vi "InitDMs_DUAL.vi"(11 "BM Flats":bool) -> (2 "IDs":i32[](array[numeric]), 3 "reference out":refnum<k7>)   [LabVIEW 2014]
uses:
  <vilib>/Utility/file.llb/Read From Spreadsheet File (DBL).vi
  <vilib>/Utility/file.llb/Read From Spreadsheet File (string).vi
  <vilib>/Analysis/Matrix/Numeric/Conversions/Array To Matrix - RA2.vi
  <vilib>/Analysis/Matrix/NI_Matrix.lvlib
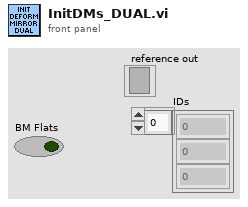
[diagram p1: front panel]
types:
  T1 = typedef "NI_Matrix.lvlib/RealMatrix.ctl" = dbl[][]
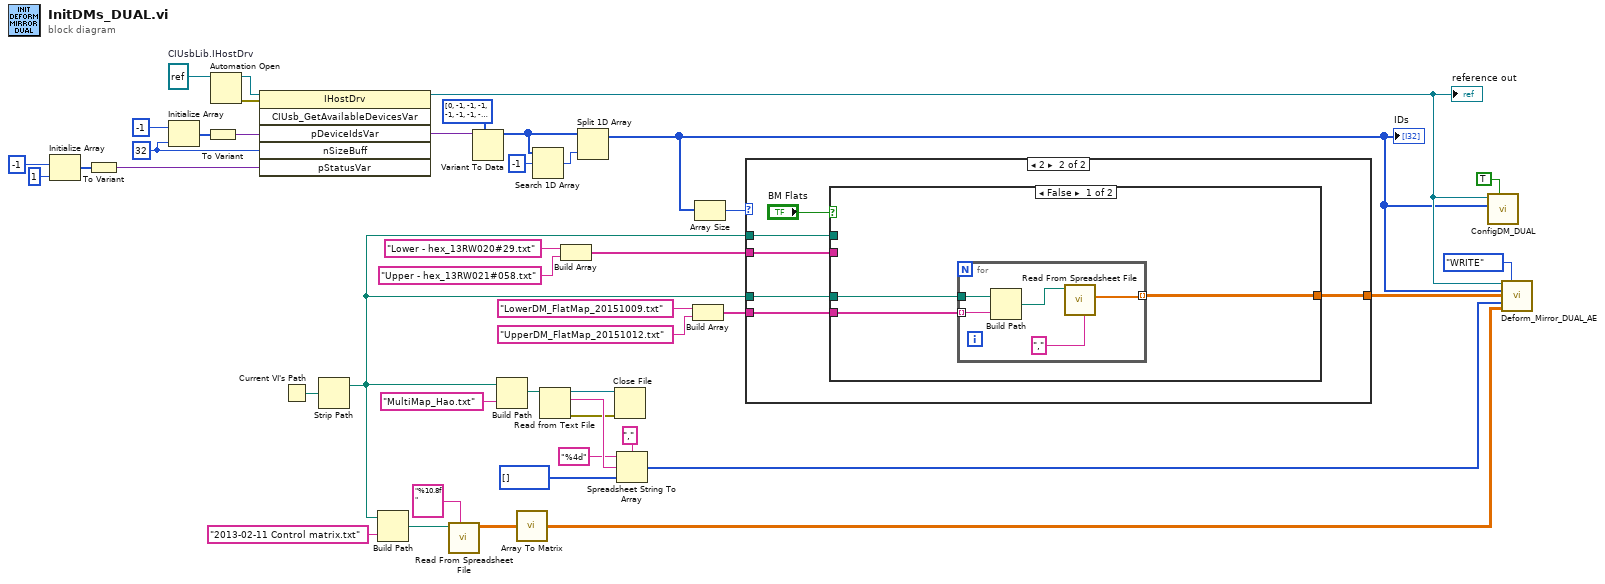
[diagram p0: block diagram]
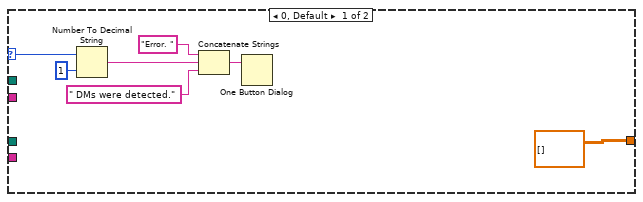
[diagram p2: hidden frame]
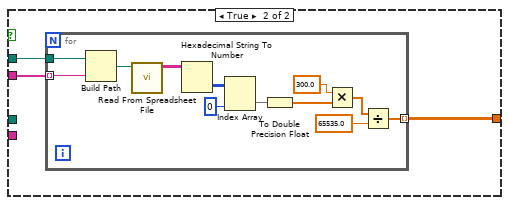
[diagram p3: hidden frame]
diagram:
  w39 = 32 ("dimension size")
  w31 = refnum<k7> refnum  # CIUsbLib.IHostDrv
  n1 = Initialize Array(-1 ("element"), 1 ("dimension size")) -> (w32:i32[])
  n2 = To Variant(anything=w32) -> (Variant=w38:variant)
  n3 = Initialize Array(-1 ("element"), w39) -> (w33:i32[])
  n4 = To Variant(anything=w33) -> (Variant=w34:variant)
  n5 = Automation Open(Automation Refnum=w31) -> (Automation Refnum=w7:refnum<k7>, error out=w36:errorcluster)  [unwired: 1 in, 2 out]
  n6 = invoke class="IHostDrv" method="CIUsb_GetAvailableDevicesVar"(reference=w7, error in=w36, "pDeviceIdsVar"=w34, "nSizeBuff"=w39, "pStatusVar"=w38) -> (reference out=w10:refnum<k7>, "pDeviceIdsVar"=w44:variant)  [unwired: 1 in, 4 out]
  "reference out" <- w10
  n7 = Current VI's Path() -> (path=w26:path)
  n8 = Strip Path(path=w26) -> (stripped path=w6:path)  [unwired: 1 out]
  n9 = Build Path(base path=w6, name or relative path="2013-02-11 Control matrix.txt") -> (appended path=w20:path)
  n10 = call-poly <vilib>:"Read From Spreadsheet File.vi"("format (%.3f)"="%10.8f", "file path (dialog if empty)"=w20) -> ("all rows"=w19:dbl[][])  [unwired: 2 in, 7 out]
  n11 = Variant To Data(type=i32[] [0, -1, -1, -1, -1, -1, -1, -1, -1, -1, -1, -1, -1, -1, -1, -1, -1, -1, -1, -1, -1, -1, -1, -1, -1, -1, -1, -1, -1, -1, -1, -1] ("pDeviceIDs"), Variant=w44) -> (data=w42:i32[])  [unwired: 1 in, 1 out]
  n12 = Build Path(base path=w6, name or relative path="MultiMap_Hao.txt") -> (appended path=w23:path)
  n13 = call-poly <vilib>:"Array To Matrix.vi"("Real 2D Array"=w19) -> ("Real Matrix"=w14:T1)
  n14 = Search 1D Array(1D array=w42, element=-1) -> (index of element=w41:i32)  [unwired: 1 in]
  n15 = Read from Text File(file (use dialog)=w23) -> (refnum out=w25:refnum<file>, text=w30:string, error out=w24:errorcluster)  [unwired: 1 in, 3 out]
  n16 = Build Array("Lower - hex_13RW020#29.txt", "Upper - hex_13RW021#058.txt" ("name or relative path")) -> (w16:string[])
  n17 = Split 1D Array(array=w42, index=w41) -> (first subarray=w9:i32[])  [unwired: 1 out]
  "IDs" <- w9
  n18 = Close File(refnum=w25, error in=w24) -> ()  [unwired: 2 out]
  n19 = Spreadsheet String To Array(delimiter (Tab)=",", format string="%4d", spreadsheet string=w30, array type (2D Dbl)=i32[] []) -> (array=w12:i32[])
  n20 = Build Array("LowerDM_FlatMap_20151009.txt" ("name or relative path"), "UpperDM_FlatMap_20151012.txt" ("name or relative path")) -> (w5:string[])
  n21 = Array Size(array=w9) -> (size(s)=w17:i32)
  n22 = case shown="2" w17 {
    selector: w17 -> [w50 _]
    tunnel: w6 -> [_ w57]
    tunnel: w16 -> [_ w56]
    tunnel: [dbl[][] [] w55] -> w15
    tunnel: w6 -> [_ w53]
    tunnel: w5 -> [_ w52]
    frame 0, Default {
      n23 = Number To Decimal String(number=w50, width (-)=i16 1) -> (decimal integer string=w48:string)
      n24 = Concatenate Strings("Error. " ("string"), w48, " DMs were detected." ("string")) -> (w45:string)
      n25 = One Button Dialog(message=w45) -> ()  [unwired: 1 in, 1 out]
    }
    frame 2 {
      n26 = case shown="False" "BM Flats" {
        tunnel: w57 -> [_ w68]
        tunnel: w56 -> [_ w67]
        tunnel: [w58 w66] -> w55
        tunnel: w53 -> [w59 _]
        tunnel: w52 -> [w60 _]
        frame False {
          n27 = for {
            tunnel: w60 -> [w64] mode=indexing
            tunnel: w59 -> [w65]
            tunnel: [w61] -> w58 mode=indexing
            n28 = Build Path(base path=w65, name or relative path=w64) -> (appended path=w62:path)
            n29 = call-poly <vilib>:"Read From Spreadsheet File.vi"("delimiter (\\t)"="," ("delimiter (\\t)"), "file path (dialog if empty)"=w62) -> ("first row"=w61:dbl[])  [unwired: 5 in, 4 out]
          }
        }
        frame True {
          n30 = for {
            tunnel: [w80] -> w66 mode=indexing
            tunnel: w68 -> [w79]
            tunnel: w67 -> [w71] mode=indexing
            n31 = Build Path(base path=w79, name or relative path=w71) -> (appended path=w78:path)
            n32 = call-poly <vilib>:"Read From Spreadsheet File.vi"("file path (dialog if empty)"=w78) -> ("all rows"=w77:string[][])  [unwired: 3 in, 7 out]
            n33 = Hexadecimal String To Number(string=w77) -> (number=w76:u32[][])  [unwired: 2 in, 1 out]
            n34 = Index Array(array=w76, index (col)=0 ("disabled index (col)")) -> (element=w74:u32[])  [unwired: 1 in]
            n35 = To Double Precision Float(number=w74) -> (double precision float=w70:dbl[])
            n36 = Multiply(x=300.0 ("y"), y=w70) -> (x*y=w73:dbl[])
            n37 = Divide(x=w73, y=65535.0) -> (x/y=w80:dbl[])
          }
        }
      }
    }
  }
  n38 = call "ConfigDM_DUAL.vi"("High Voltage"=TRUE, "Dev IDs"=w9, "Automation Refnum in"=w10) -> ()  [unwired: 7 in, 2 out]
  n39 = call "Deform_Mirror_DUAL_AE.vi"("Refnum In"=w10, "Action"=enum16{"WRITE", "READ"}."WRITE" ("Enum"), "IDs In"=w9, "Flat Files In"=w15, "Multi Map Data In"=w12, "Mode Matrix In"=w14) -> ()  [unwired: 5 in, 5 out]
